vi "OneEpoch.vi"() -> ()   [LabVIEW 2018]
uses:
  GlobalVariables/GlobalStop.vi
panel:
  in  "Stop":bool
  in  "Control Panel":T1(tab)
  in  "Filename":path=path "test.lvm"
  in  "Tolerance Range (in decimal, not %)":dbl=0.15 format="%#_13g"
  in  "Power Supply VISA resource name":refnum<visa-resource-name>
  in  "Serial Port for Arduino":refnum<visa-resource-name>="N/A"
  in  "# Successful":i16
  in  "Max Epoch":i32
  in  "Designated Garbage Pin":i32
  in  "ADC Sampling Rate":dbl=10000.0 format="%0.2f"
  in  "Delay Time (s)":dbl=0.4
  in  "Set Max Current for FP":dbl=0.25 format="%#_13g"
  in  "Initial Voltage":dbl=3.3 format="%#_13g"
  out "Actual Binary\nOutput":bool[](array[boolean])
  out "Target binary output":bool[](array[boolean])
  out "Current output":dbl
  out "Current (mA) level\nfor output pins":dbl[](array[numeric])
  out "Beginning Time Stamp":timestamp
  out "Pin Combination":i32
  out "RMSE":dbl
  out "Epoch Output":bool[][](array[boolean])
  out "All Outputs":bool[][][](array[boolean])
  out "Target Epoch":bool[][](array[boolean])
  out "Ending Time Stamp":timestamp
  out "Epochs Run":i32
  out "Successful XOR":i32
  out "Power Supply Error":string=" INSTRUCTIONS:\r\rNormal Use:  When using subVIs that incorporate the error in/error out (or error I/O) structure, place this handler where you want to inform the user of an error, typically at the end of the I/O data path, as the last action of the program.  If the error in error? is ERROR, the handler creates a message describing the error and its source.  If the type of dialog = 1 (default), the message is displayed to the user, who can only acknowedge it.  If the type = 2, the user can acknowledge the message or abort execution; aborting a program with active I/O is not recommended.  If the type = 0, no message is displayed; this is used to process the error programmatically, and the error out cluster elements are wired to individual terminals for that reason.  \r\rOther Use:\n\r\nlocal testing.  To test the error code of a subVI or function that does not have the error I/O structure, you can wire its error code and a source string to the local error code and error source inputs.  If error in error? indicates no error and error code is not equal to 0, the local code and source are substituted for the error in values, and error? is set TRUE (ERROR)."
  out "DAQ Error":string=" INSTRUCTIONS:\r\rNormal Use:  When using subVIs that incorporate the error in/error out (or error I/O) structure, place this handler where you want to inform the user of an error, typically at the end of the I/O data path, as the last action of the program.  If the error in error? is ERROR, the handler creates a message describing the error and its source.  If the type of dialog = 1 (default), the message is displayed to the user, who can only acknowedge it.  If the type = 2, the user can acknowledge the message or abort execution; aborting a program with active I/O is not recommended.  If the type = 0, no message is displayed; this is used to process the error programmatically, and the error out cluster elements are wired to individual terminals for that reason.  \r\rOther Use:\n\r\nlocal testing.  To test the error code of a subVI or function that does not have the error I/O structure, you can wire its error code and a source string to the local error code and error source inputs.  If error in error? indicates no error and error code is not equal to 0, the local code and source are substituted for the error in values, and error? is set TRUE (ERROR)."
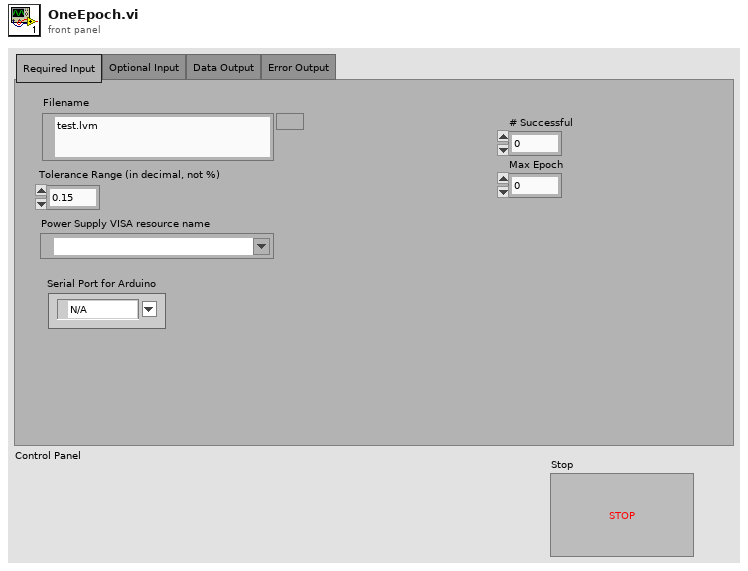
[diagram p1: front panel]
types:
  T1 = enum32{"Required Input", "Optional Input", "Data Output", "Error Output"}
  T2 = typedef "LMH-LINX.lvlib/LINX Ref.ctl" = cluster{"IO":T3, "Interface":T4, "LINX Device Config":T5}
  T3 = typedef "LMH-LINX.lvlib/Platform.ctl" = enum16{"Remote", "Local"}
  T4 = typedef "LMH-LINX.lvlib/Interface.ctl" = enum16{"Serial", "TCP"}
  T5 = typedef "LMH-LINX.lvlib/Device.lvlib/LINX Device Config.ctl" = cluster{"Interface":T4, "COM Port":refnum<visa-resource-name>, "TCP Configuration":T6, "Device Family":u8, "Device ID":u8, "Device Name":string, "TCP Ref":refnum<k5>, "Channels":T7}
  T6 = typedef "LMH-LINX.lvlib/Device.lvlib/TCP Config.ctl" = cluster{"IP Address":string, "Port":u16}
  T7 = typedef "LMH-LINX.lvlib/Channels.ctl" = cluster{"DI":u8[], "DO":u8[], "AI":u8[], "AO":u8[], "PWM":u8[], "QE":u8[], "UART":u8[], "I2C 2":u8[], "SPI":u8[], "CAN":u8[], "Servo":u8[], "AI Ref (V)":dbl, "AI Resolution (Bits)":u8, "AO Ref (V)":dbl, "AO Resolution (Bits)":u8}
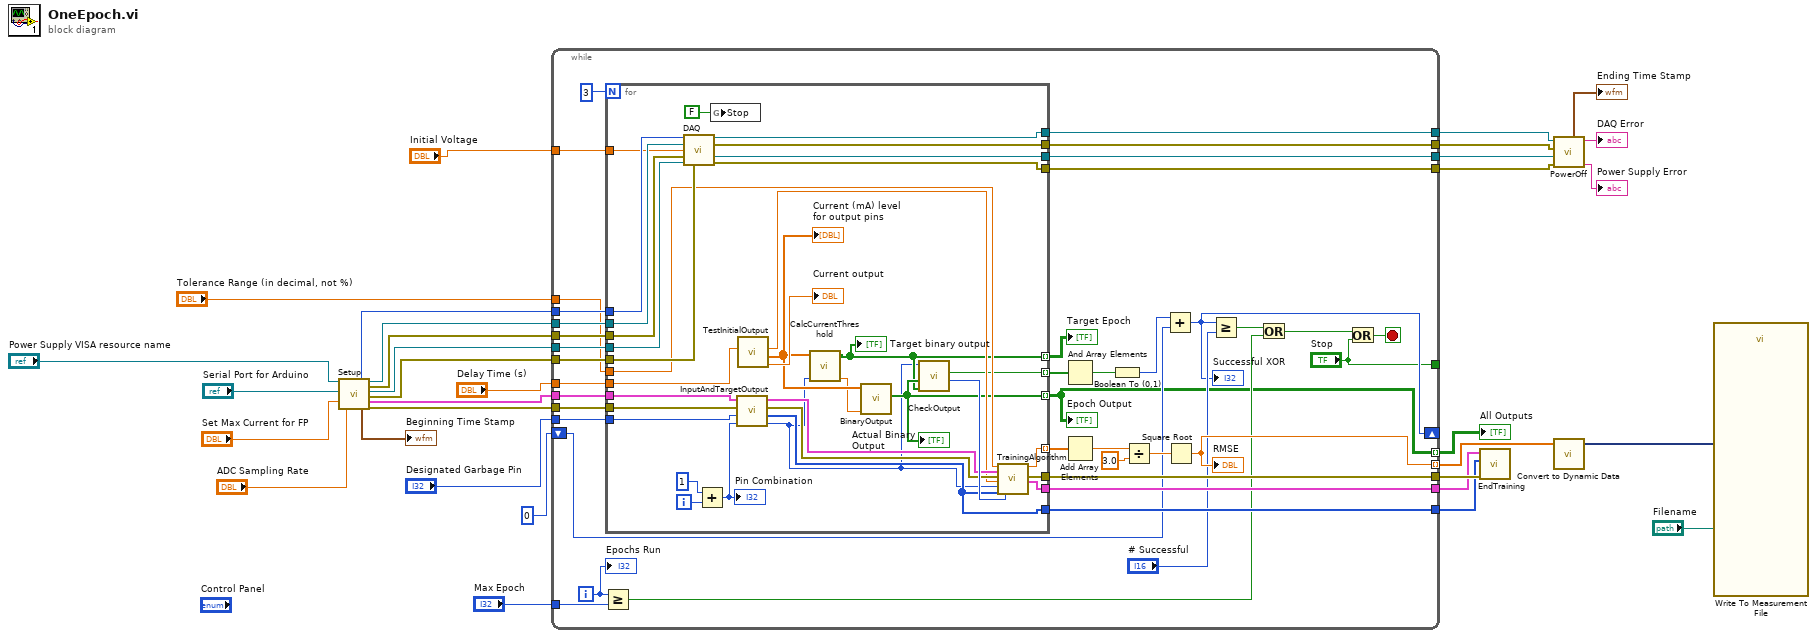
[diagram p0: block diagram]
diagram:
  n1 = call "Setup.vi"("Power Supply VISA resource name"="Power Supply VISA resource name", "Serial Port for Arduino"="Serial Port for Arduino", "Set Max Current for FP"="Set Max Current for FP", "ADC Sampling Rate"="ADC Sampling Rate") -> ("Sample Length for ADC mean 2"=w27:i32, "Beginning Time Stamp"=→"Beginning Time Stamp":timestamp, "DAQ Task Out"=w31:refnum<k21>, "DAQ Error Out"=w30:errorcluster, "VISA resource name out"=w29:refnum<visa-resource-name>, "Power Supply Error Out"=w28:errorcluster, "LINX Resource"=w26:T2, "Arduino Error Out"=w25:errorcluster)  [unwired: 8 in]
  n2 = while {
    tunnel: "Designated Garbage Pin" -> [w70]
    tunnel: w27 -> [w65]
    tunnel: "Tolerance Range (in decimal, not %)" -> [w62]
    tunnel: [w51] -> w10 mode=indexing
    tunnel: [w50] -> w8
    tunnel: "Delay Time (s)" -> [w49]
    shift-right: [w37] -> _
    shift-left: 0 -> [w40]
    tunnel: "Max Epoch" -> [w38]
    tunnel: [w36] -> w2 mode=indexing
    tunnel: w31 -> [w69]
    tunnel: [w61] -> w18
    tunnel: w30 -> [w68]
    tunnel: [w58] -> w15
    tunnel: w29 -> [w67]
    tunnel: [w59] -> w16
    tunnel: w28 -> [w66]
    tunnel: [w60] -> w17
    tunnel: w26 -> [w64]
    tunnel: [w56] -> w11
    tunnel: w25 -> [w63]
    tunnel: [w57] -> w12
    tunnel: "Initial Voltage" -> [w34]
    tunnel: ["Stop"] -> _
    i -> [w41]
    stop <- w43 stop-if-true
    n3 = Greater Or Equal?(x=w41, y=w38) -> (x >= y?=w42:bool)
    n4 = for {
      N: 3 -> [_]
      tunnel: w70 -> [w102]
      tunnel: w69 -> [w97]
      tunnel: w68 -> [w98]
      tunnel: w67 -> [w99]
      tunnel: w66 -> [w100]
      tunnel: w65 -> [w96]
      tunnel: w64 -> [w95]
      tunnel: w63 -> [w94]
      tunnel: w62 -> [w89]
      tunnel: [w88] -> w61
      tunnel: [w87] -> w60
      tunnel: [w86] -> w59
      tunnel: [w85] -> w58
      tunnel: [w84] -> w57
      tunnel: [w83] -> w56
      tunnel: [w82] -> w55 mode=indexing
      tunnel: [w81] -> w50
      tunnel: w49 -> [w80]
      tunnel: [w78] -> w48 mode=indexing
      tunnel: [w77] -> w36 mode=indexing
      tunnel: [w76] -> w35 mode=indexing
      tunnel: w34 -> [w72]
      i -> [w105]
      n5 = call "DAQ.vi"("sample length"=w96, "task/channels in"=w97, "SetVoltage"=w72, "error in"=w98, "VISA resource name out"=w99, "error out"=w100) -> ("task out"=w88:refnum<k21>, "error out 2"=w87:errorcluster, "VISA resource name out 2"=w86:refnum<visa-resource-name>, "error out 3"=w85:errorcluster)  [unwired: 6 in]
      n6 = Add(x=1, y=w105) -> (x+y=w103:i32)
      "Pin Combination" <- w103
      n7 = global write "GlobalStop.vi" "Stop"(FALSE ("Stop")) -> ()
      n8 = call "InputAndTargetOutput.vi"("Decimal Input into\nLogic Block"=w103, "Designated Garbage Pin"=w102, "Error In"=w94, "LINX Resource Input"=w95) -> ("Target Output"=w74:u32, "Arduino Digital Outputs 2"=w81:u8[], "Error Out"=w91:errorcluster, "LINX Resource Output"=w92:T2)  [unwired: 2 in, 2 out]
      n9 = call "TestInitialOutput.vi"("Delay Time (s)"=w80) -> ("Current output (mA)"=→"Current output":dbl, "Current (mA) level\nfor output pins"=w75:dbl[], "Delay Time"=w90:dbl)  [unwired: 8 in]
      "Current (mA) level\nfor output pins" <- w75
      n10 = call "CalcCurrentThreshold.vi"("Target Decimal Output"=w74, "Current of Output Pins"=w75) -> ("Current Threshold"=w73:dbl, "Target binary output"=w76:bool[])  [unwired: 7 in]
      "Target binary output" <- w76
      n11 = call "BinaryOutput.vi"("Current Threshold"=w73, "Current Level of Output Pins 2"=w75) -> ("Actual Binary\nOutput"=w77:bool[])  [unwired: 8 in, 1 out]
      "Actual Binary\nOutput" <- w77
      n12 = call "CheckOutput.vi"("Target Binary Output"=w76, "Actual Binary Output"=w77, "Expected Output Pin"=w74) -> ("Pin to Train"=w93:i32, "logical AND"=w78:bool)  [unwired: 7 in]
      n13 = call "TrainingAlgorithm.vi"("Tolerance Range (in decimal, not %)"=w89, "LINX Resource"=w92, "Error In"=w91, "Delay Time (s)"=w90, "Target \nOutput"=w74, "Arduino Digital Outputs"=w81, "Most Erroneous\nPin Index Number"=w93) -> ("[unwanted/total]^2"=w82:dbl, "Error Out"=w84:errorcluster, "LINX Resource 2"=w83:T2)  [unwired: 10 in]
    }
    "Epoch Output" <- w36
    "Target Epoch" <- w35
    n14 = And Array Elements(Boolean array=w48) -> (logical AND=w47:bool)
    n15 = Add Array Elements(numeric array=w55) -> (sum=w54:dbl)
    n16 = Boolean To (0,1)(Boolean=w47) -> (0, 1=w46:i16)
    n17 = Divide(x=w54, y=3.0) -> (x/y=w52:dbl)
    n18 = Add(x=w46, y=w40) -> (x+y=w37:i32)
    "Successful XOR" <- w37
    n19 = Square Root(x=w52) -> (sqrt(x)=w51:dbl)
    "RMSE" <- w51
    n20 = Greater Or Equal?(x=w37, y="# Successful") -> (x >= y?=w45:bool)
    n21 = Or(x=w45, y=w42) -> (x .or. y?=w44:bool)
    n22 = Or(x=w44, y="Stop") -> (x .or. y?=w43:bool)
    "Epochs Run" <- w41
  }
  "All Outputs" <- w2
  n23 = call "EndTraining.vi"("Error In"=w12, "DO Channels"=w8, "LINX Resource"=w11) -> ()  [unwired: 9 in]
  n24 = call "PowerOff.vi"("Power Supply Error IN"=w15, "VISA resource name"=w16, "DAQ Error In"=w17, "DAQ Channels"=w18) -> ("Power Supply Error"=→"Power Supply Error":string, "DAQ Error"=→"DAQ Error":string, "Ending Time Stamp 2"=→"Ending Time Stamp":timestamp)  [unwired: 5 in]
  n25 = call "Convert to Dynamic Data"("Array"=w10) -> ("Dynamic Data Type"=w4:dynamicdata)  [unwired: 3 in]
  n26 = call "Write To Measurement File"("Signals"=w4, "Filename"="Filename") -> ()  [unwired: 15 in, 3 out]
